vi "ExSub3strip.vi"(2 "error in (no error)":errorcluster, 3 "Camera Handle":u32) -> (0 "error out":errorcluster, 1 "Camera Handle":u32)   [LabVIEW 2010]
panel:
  out "region 3 y":u32
  out "region 2 y":u32
  out "region 1 y":u32
  # "ExSub3Strip:\nThis Sub-VI takes 3 strips from a CCD and\nequally spaces the strips so that one is \nin the top 1/3rd of the CCD, one is in\nthe center, and the last is in the bottom \n1/3rd of the CCD. It then programs up \nthe camera with these 3 ROIs"
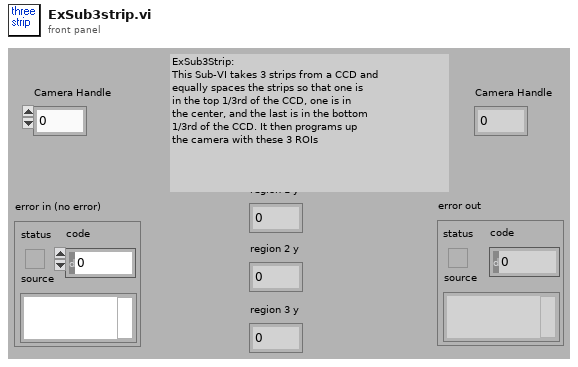
[diagram p1: front panel]
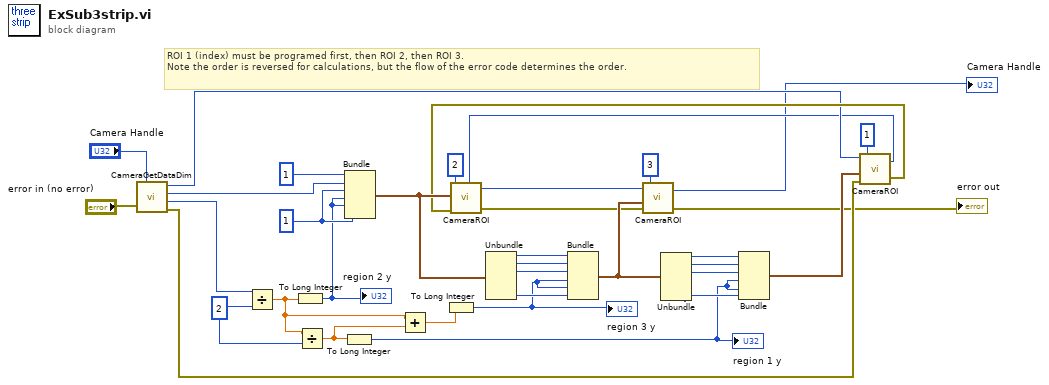
[diagram p0: block diagram]
diagram:
  w29 = 2
  w33 = 1
  # "ROI 1 (index) must be programed first, then ROI 2, then ROI 3.\nNote the order is reversed for calculations, but the flow of the error code determines the order."
  n1 = call <userlib>:"CameraGetDataDim.vi"("Camera Handle"="Camera Handle", "error in"="error in (no error)") -> ("Camera Handle"=w9:u32, "Xdim"=w24:u32, "Ydim"=w30:u32, "error out"=w12:errorcluster)
  n2 = Divide(x=w30, y=w29) -> (x/y=w28:dbl)
  n3 = To Long Integer(number=w28) -> (32bit integer=w1:i32)
  "region 2 y" <- w1
  n4 = Divide(x=w28, y=w29) -> (x/y=w27:dbl)
  n5 = To Long Integer(number=w27) -> (32bit integer=w3:i32)
  "region 1 y" <- w3
  n6 = Bundle(1, "Xdim"=w24, w33, w1, w1, w33) -> (w11:cluster{i32, "Xdim":u32, i32, i32, i32, i32})  [unwired: 1 in]
  n7 = Add(x=w28, y=w27) -> (x+y=w26:dbl)
  n8 = To Long Integer(number=w26) -> (32bit integer=w2:i32)
  "region 3 y" <- w2
  n9 = Unbundle(w11) -> (w23:i32, "Xdim"=w22:u32, w21:i32, w20:i32)  [unwired: 2 out]
  n10 = Bundle(w23, "Xdim"=w22, w21, w2, w2, w20) -> (w19:cluster{i32, "Xdim":u32, i32, i32, i32, i32})  [unwired: 1 in]
  n11 = Unbundle(w19) -> (w18:i32, "Xdim"=w17:u32, w16:i32, w15:i32)  [unwired: 2 out]
  n12 = Bundle(w18, "Xdim"=w17, w16, w3, w3, w15) -> (w14:cluster{i32, "Xdim":u32, i32, i32, i32, i32})  [unwired: 1 in]
  n13 = call <userlib>:"CameraROI.vi"("error in"=w12, "ROI Params"=w14, "ROI Index"=1, "Camera Handle"=w9) -> ("error out"=w10:errorcluster, "Camera Handle"=w8:u32)
  n14 = call <userlib>:"CameraROI.vi"("error in"=w10, "ROI Params"=w11, "ROI Index"=2, "Camera Handle"=w8) -> ("error out"=w6:errorcluster, "Camera Handle"=w7:u32)
  n15 = call <userlib>:"CameraROI.vi"("error in"=w6, "ROI Params"=w19, "ROI Index"=3, "Camera Handle"=w7) -> ("error out"=→"error out":errorcluster, "Camera Handle"=→"Camera Handle":u32)
